vi "Add Data Channels.vi"(7 "# Elements":u32, 8 "Error In":errorcluster, 9 "Units":string, 10 "Default Value":dbl, 11 "Data Array Section Refnum In":T1 format="%.0x") -> (0 "Error Out":errorcluster)   [LabVIEW 2018, in "Instrument Addon System Explorer.lvlib"]
doc: "Adds the specified number of Data Array Channels under the Data Array section provided as input.\n\nInput:\nData Array Section Refnum In: reference to the Data Array section under which the channels are about to be added.\nDefault Value: represents the default value of the channel.\nUnits: represents the units of the default value (e.g. ms).\n# Elements: the number of desired channels.\n\nOutput:\nn/a"
uses:
  Instrument Addon System Explorer.lvlib
  <vilib>/NI Veristand/Custom Device API/Custom Device Item Ref.ctl
  APIs/Scripting API/TypeDefs/Array Element.ctl
  Addon Shared/SubVIs/Constants.vi
  APIs/Scripting API/Instrument Addon Scripting API.lvlib
  <vilib>/NI Veristand/Custom Device API/Custom Device API.lvlib
  Addon Shared/Instrument Addon Shared.lvlib
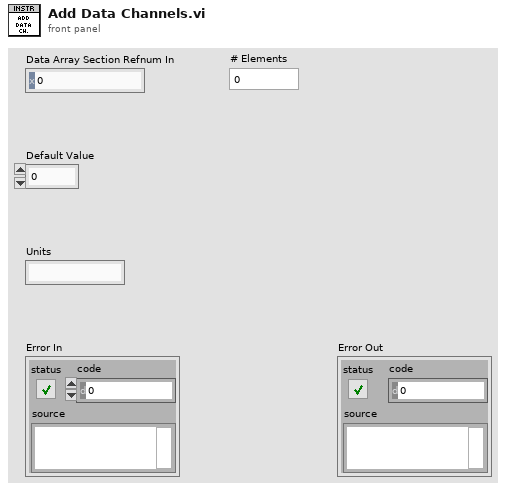
[diagram p1: front panel]
types:
  T1 = typedef "Custom Device API.lvlib/Custom Device Item Ref.ctl" = u64
  T2 = typedef "Instrument Addon Scripting API.lvlib/Array Element.ctl" = cluster{"Name":string, "Default Value":dbl, "Units":string}
  T3 = typedef "Custom Device API.lvlib/Custom Device Item Info.ctl" = cluster{"Name":string, "Is Channel":bool, "GUID":string, "Is Waveform":bool}
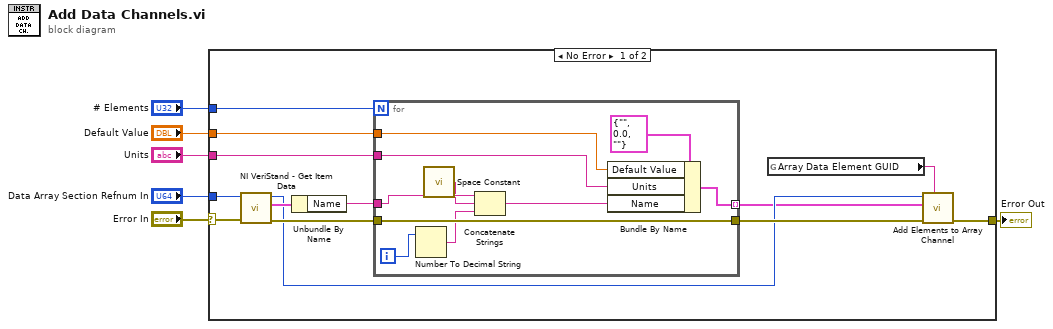
[diagram p0: block diagram]
diagram:
  n1 = case shown="No Error" "Error In" {
    selector: "Error In" -> [w15 w30]
    tunnel: "Units" -> [w19 _]
    tunnel: "Default Value" -> [w18 _]
    tunnel: [w13 w30] -> w4
    tunnel: "Data Array Section Refnum In" -> [w16 _]
    tunnel: "# Elements" -> [w12 _]
    frame No Error {
      n2 = call <vilib>:"NI VeriStand - Get Item Data.vi"("error in (no error)"=w15, "Item Ref in"=w16) -> ("error out"=w11:errorcluster, "Item Info"=w17:T3, "Item Ref out"=w9:T1)  [unwired: 7 out]
      n3 = Unbundle By Name(w17) -> ("Name"=w14:string)
      n4 = for {
        N: w12 -> [_]
        tunnel: w19 -> [w29]
        tunnel: w18 -> [w28]
        tunnel: w14 -> [w23]
        tunnel: w11 -> [w26]
        tunnel: [w26] -> w10
        tunnel: [w25] -> w8 mode=indexing
        i -> [w24]
        n5 = Number To Decimal String(number=w24) -> (decimal integer string=w21:string)  [unwired: 1 in]
        n6 = call <vilib>:"Space Constant.vi"() -> ("String"=w22:string)
        n7 = Concatenate Strings(w23, w22, w21) -> (w20:string)
        n8 = Bundle By Name(cluster=T2 {"Name"="", "Default Value"=0.0, "Units"=""} ("Array Element"), "Default Value"=w28, "Units"=w29, "Name"=w20) -> (w25:T2)
      }
      n9 = global read "Constants.vi" "Array Data Element GUID"() -> (w7:string)
      n10 = call "Add Elements to Array Channel.vi"("array element GUID"=w7, "error in (no error)"=w10, "array elements"=w8, "array refnum in"=w9) -> ("error out"=w13:errorcluster)  [unwired: 5 in, 2 out]
    }
    frame Error {
    }
  }
  "Error Out" <- w4
